vi "Read Button Properties.vi"(8 "error in (no error)":errorcluster, 11 "RunTimeButton in":refnum<class "RunTimeButton.lvclass">) -> (0 "error out":errorcluster, 2 "Button":T1, 3 "RunTimeButton out":refnum<class "RunTimeButton.lvclass">)   [LabVIEW 2019, in "RunTimeButton.lvclass"]
uses:
  RunTimeButton.lvclass
  XML Controls/ButtonLists Properties.ctl
  XML Controls/Path Cluster.ctl
  XML Controls/Button Type.ctl
  XML Controls/Dependency Properties.ctl
  RunTimeButton.lvclass/RunTimeButton.ctl
  VeriStand Custom Device XML Parser.lvlib
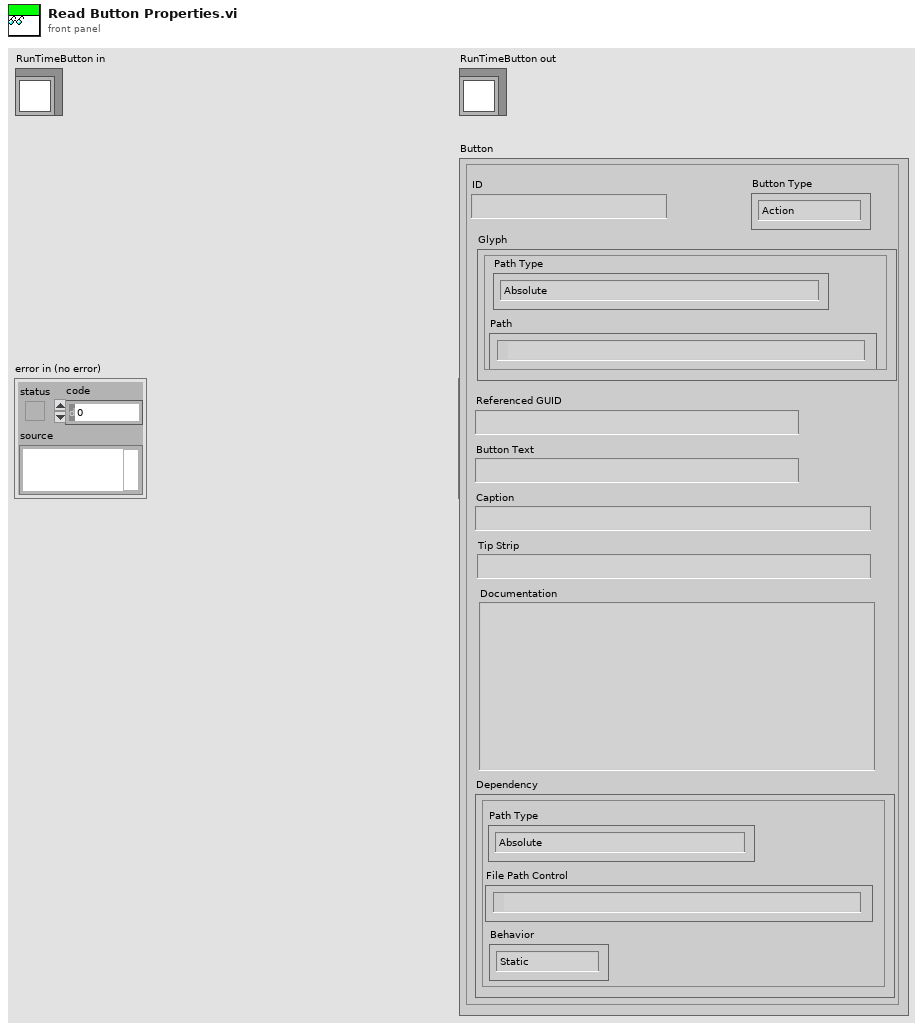
[diagram p1: front panel]
types:
  T1 = typedef "VeriStand Custom Device XML Parser.lvlib/ButtonLists Properties.ctl" = cluster{"ID":string, "Glyph":T2, "Button Type":T3, "Referenced GUID":string, "Button Text":string, "Caption":string, "Tip Strip":string, "Documentation":string, "Dependency":T4}
  T2 = typedef "VeriStand Custom Device XML Parser.lvlib/Path Cluster.ctl" = cluster{"Path":path, "Path Type":enum16{"Absolute", "To Base", "To Common Doc Dir", "To Application Data Dir"}}
  T3 = typedef "VeriStand Custom Device XML Parser.lvlib/Button Type.ctl" = enum16{"Action", "Dialog", "Page", "Notification", "Separator"}
  T4 = typedef "VeriStand Custom Device XML Parser.lvlib/Dependency Properties.ctl" = cluster{"File Path Control":path, "Path Type":enum16{"Absolute", "To Base", "To Common Doc Dir", "To Application Data Dir"}, "Behavior":enum16{"Static", "Dynamic"}}
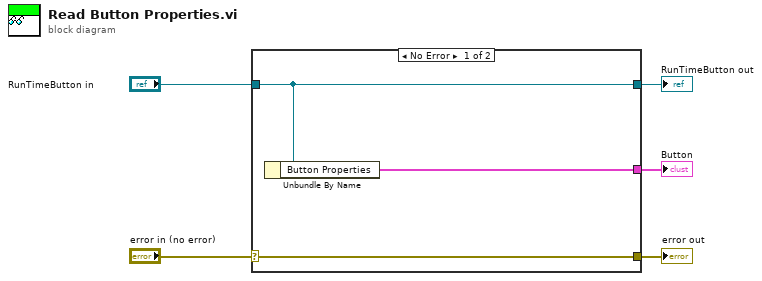
[diagram p0: block diagram]
diagram:
  n1 = case shown="No Error" "error in (no error)" {
    selector: "error in (no error)" -> [w8 w9]
    tunnel: [w8 w9] -> w4
    tunnel: [w7 w10] -> w2
    tunnel: "RunTimeButton in" -> [w7 w10]
    tunnel: [w6 _] -> w1
    frame No Error {
      n2 = Unbundle By Name(w7) -> ("Button Properties"=w6:T1)
    }
    frame Error {
    }
  }
  "error out" <- w4
  "RunTimeButton out" <- w2
  "Button" <- w1
